vi "Is Type.vi"(11 "OptionalType in":refnum<class "OptionalType.lvclass">) -> ()   [LabVIEW 2017, in "OptionalType.lvclass"]
uses:
  OptionalType.lvclass
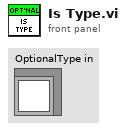
[diagram p1: front panel]
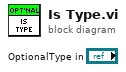
[diagram p0: block diagram]
diagram:
